vi "Drive PID.vi"(11 "Process Variable":dbl format="%.2f") -> (3 "Output":dbl format="%.2f")   [LabVIEW 2012]
uses:
  <vilib>/addons/control/pid/pid.llb/PID (DBL).vi
  Begin/Global Variables.vi
  <vilib>/addons/control/pid/NI_PID_pid.lvlib
panel:
  # "Used more than once at a time,\ntherefore VI Properties > Execution\nshould be Preallocated clone reentrant"
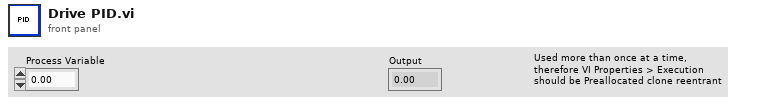
[diagram p1: front panel]
types:
  T1 = cluster{"proportional gain (Kc)":dbl, "integral time (Ti, min)":dbl, "derivative time (Td, min)":dbl}
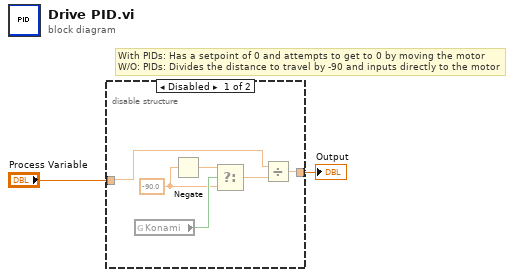
[diagram p0: block diagram]
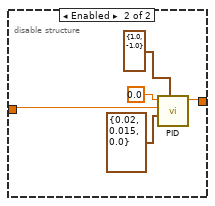
[diagram p2: hidden frame]
diagram:
  # "With PIDs: Has a setpoint of 0 and attempts to get to 0 by moving the motor\nW/O: PIDs: Divides the distance to travel by -90 and inputs directly to the motor"
  n1 = disable-structure shown="Disabled" {
    disable-tunnel: "Process Variable" -> [w3 w10]
    disable-tunnel: [w4 w9] -> w1
    frame Disabled {
      w5 = -90.0 ("y")
      n2 = global read "Global Variables.vi" "Konami"() -> (w8:bool)
      n3 = Negate(x=w5) -> (-x=w6:dbl)
      n4 = Select(t=w6, s=w8, f=w5) -> (s? t:f=w7:dbl)
      n5 = Divide(x=w3, y=w7) -> (x/y=w4:dbl)
    }
    frame Enabled {
      n6 = call-poly <vilib>:"PID.vi"("output range"=cluster{"output high":dbl, "output low":dbl} {"output high"=1.0, "output low"=-1.0}, "PID gains"=T1 {"proportional gain (Kc)"=0.02, "integral time (Ti, min)"=0.015, "derivative time (Td, min)"=0.0}, "process variable"=w10, "setpoint"=0.0) -> ("output"=w9:dbl)  [unwired: 6 in, 1 out]
    }
  }
  "Output" <- w1
